vi "Search DBL Array.vi"(10 "Array":dbl[](array[numeric])=[3.814697265625, 500000.0, 256.0, 512.0] format="%.6f", 11 "Target":dbl format="%.8f") -> (2 "Actual Value":dbl format="%.2f", 3 "Row Index":i32)   [LabVIEW 2021]
panel:
  # "Uses bisection to find the index of the row\nwhere the value is the closest to the specified\ntarget value.\n\nInput array must be sorted in ascending order."
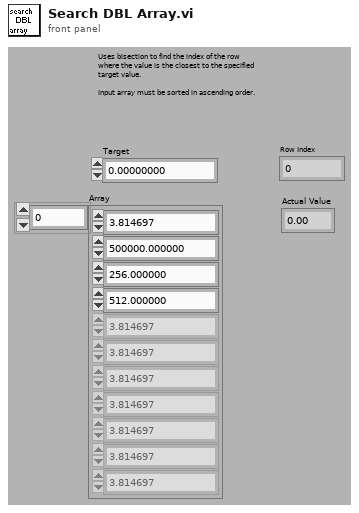
[diagram p1: front panel]
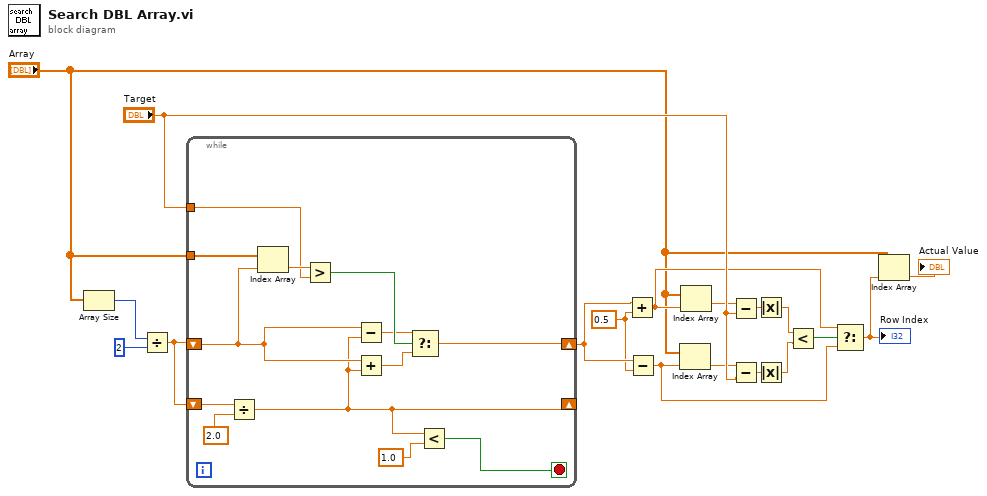
[diagram p0: block diagram]
diagram:
  w14 = 0.5 ("y")
  n1 = Array Size(array="Array") -> (size(s)=w17:i32)
  n2 = Divide(x=w17, y=2) -> (x/y=w16:dbl)
  n3 = while {
    shift-right: [w24] -> w15
    shift-left: w16 -> [w22]
    tunnel: "Array" -> [w31]
    tunnel: "Target" -> [w29]
    shift-right: [w21] -> _
    shift-left: w16 -> [w27]
    stop <- w19 stop-if-true
    n4 = Divide(x=w27, y=2.0) -> (x/y=w21:dbl)
    n5 = Index Array(array=w31, index=w22) -> (element=w30:dbl)
    n6 = Greater?(x=w30, y=w29) -> (0:w26:bool)
    n7 = Subtract(x=w22, y=w21) -> (x-y=w25:dbl)
    n8 = Add(x=w22, y=w21) -> (x+y=w23:dbl)
    n9 = Select(t=w25, s=w26, f=w23) -> (s? t:f=w24:dbl)
    n10 = Less?(x=w21, y=1.0) -> (x < y?=w19:bool)
  }
  n11 = Add(x=w15, y=w14) -> (x+y=w10:dbl)
  n12 = Subtract(x=w15, y=w14) -> (x-y=w8:dbl)
  n13 = Index Array(array="Array", index=w8) -> (element=w12:dbl)
  n14 = Index Array(array="Array", index=w10) -> (element=w11:dbl)
  n15 = Subtract(x=w11, y="Target") -> (x-y=w7:dbl)
  n16 = Subtract(x=w12, y="Target") -> (x-y=w5:dbl)
  n17 = Absolute Value(x=w7) -> (abs(x)=w6:dbl)
  n18 = Absolute Value(x=w5) -> (abs(x)=w4:dbl)
  n19 = Less?(x=w6, y=w4) -> (x < y?=w9:bool)
  n20 = Select(t=w10, s=w9, f=w8) -> (s? t:f=w3:dbl)
  "Row Index" <- w3
  n21 = Index Array(array="Array", index=w3) -> (element=→"Actual Value":dbl)
